vi "Img Data to Bitmap.vi"(10 "threshold":u8=10, 11 "image data":T1) -> (3 "bitmap":u32[][](array[numeric]))   [LabVIEW 2018, in "Image Process.lvclass"]
uses:
  Image Process.lvclass
  <vilib>/picture/picture.llb/imagedata.ctl
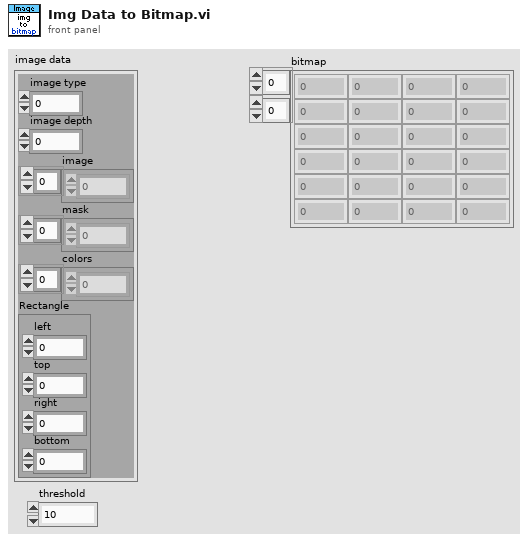
[diagram p1: front panel]
types:
  T1 = typedef "imagedata.ctl" = cluster{"image type":i32, "image depth":i32, "image":u8[], "mask":u8[], "colors":u32[], "Rectangle":cluster{"left":i16, "top":i16, "right":i16, "bottom":i16}}
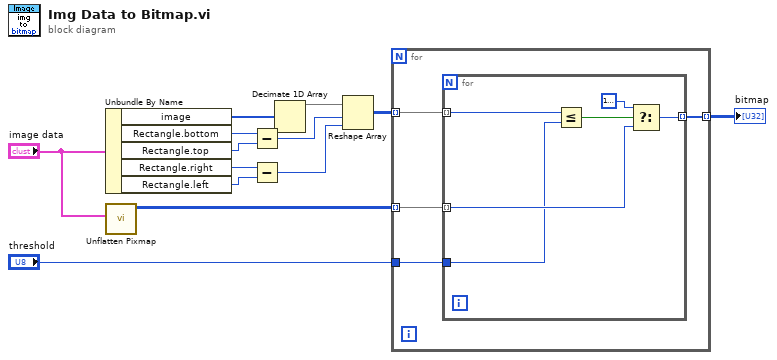
[diagram p0: block diagram]
diagram:
  n1 = Unbundle By Name("image data") -> ("image"=w9:u8[], "Rectangle.bottom"=w13:i16, "Rectangle.top"=w12:i16, "Rectangle.right"=w11:i16, "Rectangle.left"=w10:i16)
  n2 = call <vilib>:"Unflatten Pixmap.vi"("image data"="image data") -> ("24-bit pixmap"=w4:u32[][])  [unwired: 4 in, 6 out]
  n3 = Subtract(x=w13, y=w12) -> (x-y=w7:i16)
  n4 = Subtract(x=w11, y=w10) -> (x-y=w6:i16)
  n5 = Decimate 1D Array(w9) -> (w8:u8[])  [unwired: 3 out]
  n6 = Reshape Array(w8, w7, w6) -> (w5:u8[][])
  n7 = for {
    tunnel: w5 -> [w17] mode=indexing
    tunnel: w4 -> [w16] mode=indexing
    tunnel: [w15] -> w3 mode=indexing
    tunnel: "threshold" -> [w14]
    n8 = for {
      tunnel: w17 -> [w20] mode=indexing
      tunnel: w16 -> [w22] mode=indexing
      tunnel: [w21] -> w15 mode=indexing
      tunnel: w14 -> [w18]
      n9 = Less Or Equal?(x=w20, y=w18) -> (x <= y?=w19:bool)
      n10 = Select(t=u32 16777216, s=w19, f=w22) -> (s? t:f=w21:u32)
    }
  }
  "bitmap" <- w3
